vi "__power_difference.vi"(1 "Power Low dBm":dbl[](array[numeric]), 2 "Power High dBm":dbl[](array[numeric])) -> (0 "Power Difference dBm":dbl[](array[numeric]))   [LabVIEW 2013]
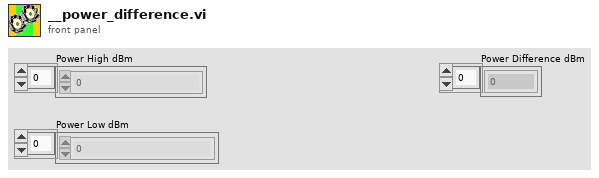
[diagram p1: front panel]
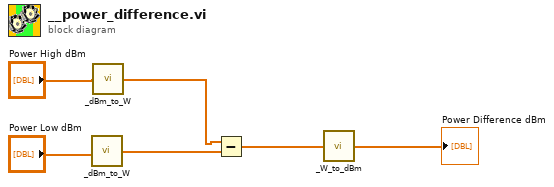
[diagram p0: block diagram]
diagram:
  n1 = call "_dBm_to_W.vi"("Power dBm"="Power Low dBm") -> ("Power W"=w1:dbl[])
  n2 = call "_dBm_to_W.vi"("Power dBm"="Power High dBm") -> ("Power W"=w2:dbl[])
  n3 = Subtract(x=w2, y=w1) -> (x-y=w4:dbl[])
  n4 = call "_W_to_dBm.vi"("Power W"=w4) -> ("Power dBm"=→"Power Difference dBm":dbl[])
